vi "tls http connection handler.vi"(8 "http responder":refnum<class "https responder.lvclass">, 9 "remote address":string, 10 "basic HTTP handler dataset":refnum<class "HTTPS handler dataset.lvclass">, 11 "connection":refnum<k5>) -> ()   [LabVIEW 2016, in "Basic HTTPS server.lvclass"]
uses:
  Basic HTTPS server.lvclass
  HTTP responder/https responder.lvclass
  HTTP handler dataset/HTTPS handler dataset.lvclass
  HTTP handler dataset/HTTPS handler dataset.lvclass/HTTPS handler dataset.ctl
  http request.ctl
  http method.ctl
  HTTP headers/http header data.ctl
  https handler parse state.ctl
  HTTP headers/http headers.lvlib
  lvlibtls/socket connection/lvlibretls connection.lvclass
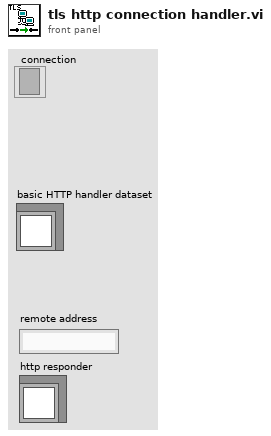
[diagram p1: front panel]
types:
  T1 = typedef "Basic HTTPS server.lvclass/http server info.ctl" = cluster{"port":u16}
  T2 = typedef "Basic HTTPS server.lvclass/http server properties.ctl" = cluster{"max url size":i32, "max header":i32, "timeout ms":i32, "max data size":i32}
  T3 = typedef "Basic HTTPS server.lvclass/https handler parse state.ctl" = enum16{"function", "headers", "data", "process"}
  T4 = typedef "Basic HTTPS server.lvclass/http request.ctl" = cluster{"type":T5, "remote address":string, "method":string, "url":string, "version":string, "headers":T6, "data":string}
  T5 = typedef "Basic HTTPS server.lvclass/http method.ctl" = enum16{"application", "error", "upgrade"}
  T6 = typedef "http headers.lvlib/http header data.ctl" = cluster{"lookup":variant}
  T7 = typedef "Basic HTTPS server.lvclass/http response.ctl" = cluster{"reason code":u16, "status string":string, "headers":T6, "cookies":string[], "data":string}
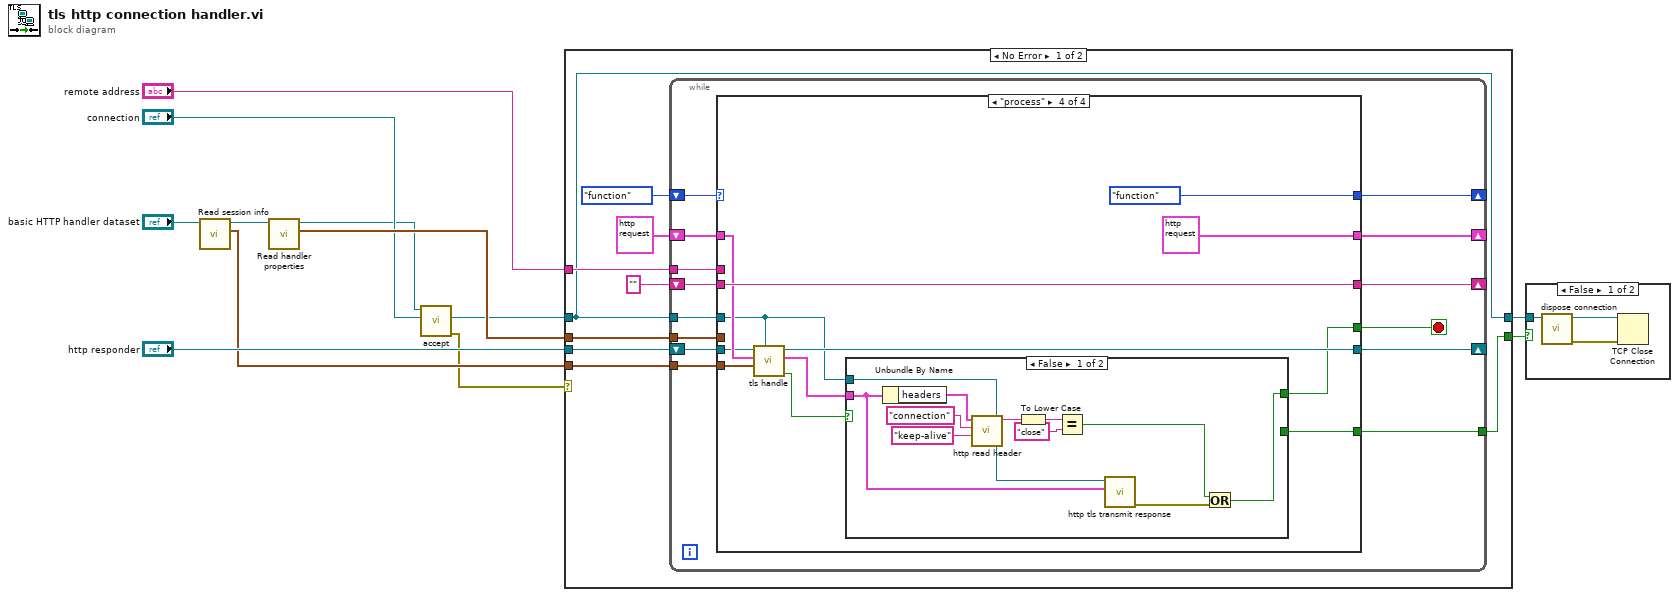
[diagram p0: block diagram]
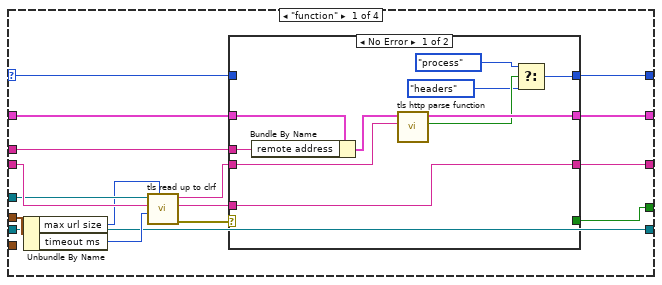
[diagram p2: hidden frame]
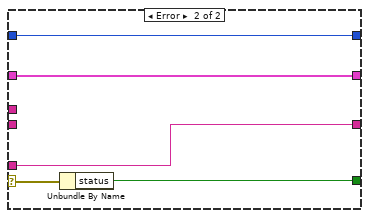
[diagram p3: hidden frame]
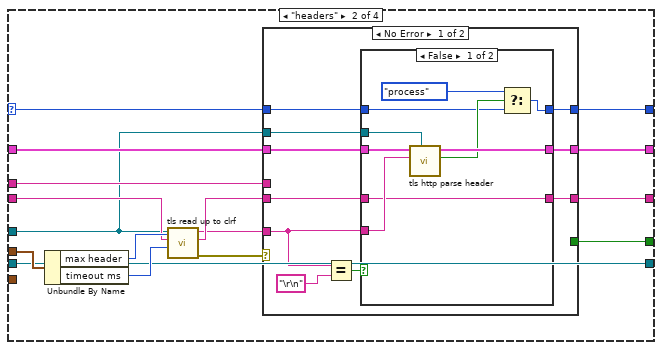
[diagram p4: hidden frame]
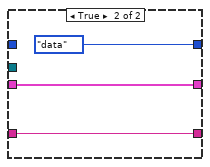
[diagram p5: hidden frame]
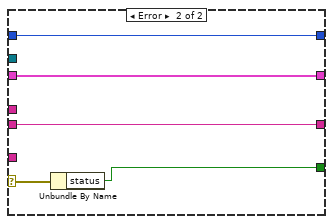
[diagram p6: hidden frame]
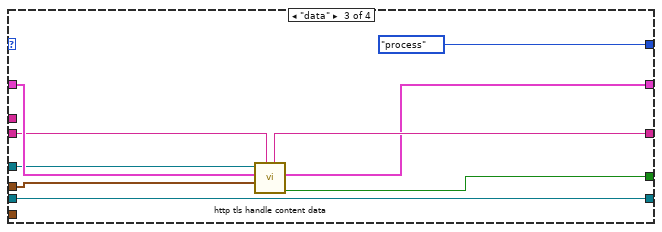
[diagram p7: hidden frame]
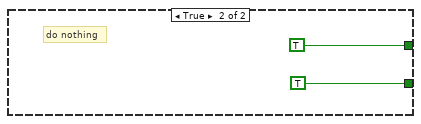
[diagram p8: hidden frame]
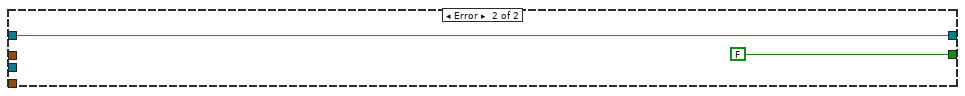
[diagram p9: hidden frame]
diagram:
  n1 = call "Read session info.vi"("basic HTTP handler dataset in"="basic HTTP handler dataset") -> ("server information"=w7:T1, "basic HTTP handler dataset out"=w9:refnum<class "HTTPS handler dataset.lvclass">)  [unwired: 9 in]
  n2 = call "Read handler properties.vi"("basic HTTP handler dataset in"=w9) -> ("server properties"=w10:T2, "basic HTTP handler dataset out"=w1:refnum<class "HTTPS handler dataset.lvclass">)  [unwired: 9 in]
  n3 = call "accept.vi"("connection ID"="connection", "TLS HTTP handler dataset in"=w1) -> ("error out"=w6:errorcluster, "lvlibretls connection"=w5:refnum<class "lvlibretls connection.lvclass">)  [unwired: 8 in]
  n4 = case shown="No Error" w6 {
    tunnel: w5 -> [w17 w145]
    tunnel: "remote address" -> [w21 _]
    tunnel: w10 -> [w19 _]
    tunnel: "http responder" -> [w14 _]
    tunnel: w7 -> [w15 _]
    tunnel: [w17 w145] -> w3
    tunnel: [w13 FALSE] -> w2
    frame No Error {
      n5 = while {
        tunnel: w17 -> [w28]
        shift-right: [w34] -> _
        shift-left: T4 {"type"=enum."application", "remote address"="", "method"="", "url"="", "version"="", "headers"={"lookup"=variant}, "data"=""} ("application request") -> [w35]
        shift-right: [w33] -> _
        shift-left: https_handler_parse_state."function" -> [w30]
        tunnel: w21 -> [w32]
        tunnel: w19 -> [w31]
        shift-right: [w26] -> _
        shift-left: "" -> [w27]
        tunnel: w15 -> [w25]
        shift-right: [w23] -> _
        shift-left: w14 -> [w24]
        tunnel: [w22] -> w13
        stop <- w29 stop-if-true
        n6 = case shown="\"process\"" w30 {
          selector: w30 -> [w47 w78 _ _]
          tunnel: w35 -> [w51 w82 w117 w126]
          tunnel: [w50 w81 w111 T4 {"type"=enum."application", "remote address"="", "method"="", "url"="", "version"="", "headers"={"lookup"=variant}, "data"=""} ("application request")] -> w34
          tunnel: w28 -> [w43 w68 w116 w122]
          tunnel: [w49 w80 https_handler_parse_state."process" https_handler_parse_state."function"] -> w33
          tunnel: w32 -> [w48 w79 _ _]
          tunnel: w31 -> [w46 w77 w118 _]
          tunnel: [w36 w67 w110 w120] -> w29
          tunnel: w27 -> [w45 w73 w115 w128]
          tunnel: [w38 w76 w114 w128] -> w26
          tunnel: w25 -> [_ _ _ w127]
          tunnel: w24 -> [w37 w69 w112 w125]
          tunnel: [w37 w69 w112 w124] -> w23
          tunnel: [_ _ _ w119] -> w22
          frame "function" {
            n7 = Unbundle By Name(w46) -> ("max url size"=w41:i32, "timeout ms"=w42:i32)
            n8 = call "tls read up to clrf.vi"("max size"=w41, "timeout ms"=w42, "buffer in"=w45, "lvlibretls connection in"=w43) -> ("error out"=w40:errorcluster, "buffer out"=w39:string, "line out"=w44:string)  [unwired: 5 in]
            n9 = case shown="No Error" w40 {
              selector: w40 -> [_ w65]
              tunnel: w51 -> [w60 w66]
              tunnel: [w61 w66] -> w50
              tunnel: w39 -> [w57 w63]
              tunnel: w47 -> [_ w64]
              tunnel: [w52 w64] -> w49
              tunnel: w48 -> [w59 _]
              tunnel: w44 -> [w56 _]
              tunnel: [w57 w63] -> w38
              tunnel: [_ w62] -> w36
              frame No Error {
                n10 = Bundle By Name(cluster=w60, "remote address"=w59) -> (w58:T4)
                n11 = call "tls http parse function.vi"("data in"=w56, "application request in"=w58) -> ("error"=w55:bool, "application request out"=w61:T4)  [unwired: 8 in]
                n12 = Select(t=https_handler_parse_state."process", s=w55, f=https_handler_parse_state."headers") -> (s? t:f=w52:T3)
              }
              frame Error {
                n13 = Unbundle By Name(w65) -> ("status"=w62:bool)
              }
            }
          }
          frame "headers" {
            n14 = Unbundle By Name(w77) -> ("max header"=w75:i32, "timeout ms"=w74:i32)
            n15 = call "tls read up to clrf.vi"("max size"=w75, "timeout ms"=w74, "buffer in"=w73, "lvlibretls connection in"=w68) -> ("error out"=w70:errorcluster, "buffer out"=w72:string, "line out"=w71:string)  [unwired: 5 in]
            n16 = case shown="No Error" w70 {
              selector: w70 -> [_ w108]
              tunnel: w82 -> [w88 w109]
              tunnel: [w89 w109] -> w81
              tunnel: w71 -> [w91 _]
              tunnel: w78 -> [w92 w107]
              tunnel: [w90 w107] -> w80
              tunnel: w79 -> [_ _]
              tunnel: w72 -> [w84 w106]
              tunnel: [w85 w106] -> w76
              tunnel: w68 -> [w83 _]
              tunnel: [_ w105] -> w67
              frame No Error {
                n17 = Equal?(x=w91, y="\r\n" ("x")) -> (x = y?=w86:bool)
                n18 = case shown="False" w86 {
                  tunnel: w91 -> [w101 _]
                  tunnel: w88 -> [w100 w104]
                  tunnel: [w99 w104] -> w89
                  tunnel: w92 -> [w96 _]
                  tunnel: [w95 https_handler_parse_state."data"] -> w90
                  tunnel: [w98 w103] -> w85
                  tunnel: w84 -> [w98 w103]
                  tunnel: w83 -> [w93 _]
                  frame False {
                    n19 = call "tls http parse header.vi"("lvlibretls connection in"=w93, "data in"=w101, "application request"=w100) -> ("abort"=w97:bool, "application request out"=w99:T4)  [unwired: 7 in]
                    n20 = Select(t=https_handler_parse_state."process", s=w97, f=w96) -> (s? t:f=w95:T3)
                  }
                  frame True {
                  }
                }
              }
              frame Error {
                n21 = Unbundle By Name(w108) -> ("status"=w105:bool)
              }
            }
          }
          frame "data" {
            n22 = call "http tls handle content data.vi"("buffer in"=w115, "server properties"=w118, "application request"=w117, "lvlibretls connection in"=w116) -> ("connection error"=w110:bool, "application request out"=w111:T4, "buffer out"=w114:string)  [unwired: 5 in]
          }
          frame "process" {
            n23 = call "tls handle.vi"("lvlibretls connection"=w122, "server information"=w127, "application request in"=w126, "http responder in"=w125) -> ("connection upgrade"=w121:bool, "response"=w123:T7, "http responder out"=w124:refnum<class "https responder.lvclass">)  [unwired: 5 in]
            n24 = case shown="False" w121 {
              tunnel: w123 -> [w135 _]
              tunnel: w122 -> [w136 _]
              tunnel: [w132 TRUE] -> w120
              tunnel: [_ TRUE] -> w119
              frame False {
                n25 = Unbundle By Name(w135) -> ("headers"=w140:T6)
                n26 = call "http read header.vi"("default value"="keep-alive", "header field name"="connection" ("name"), "headers"=w140) -> ("value"=w137:string)  [unwired: 7 in, 1 out]
                n27 = To Lower Case(string=w137) -> (all lower case string=w131:string)
                n28 = Equal?(x=w131, y="close" ("name")) -> (x = y?=w133:bool)
                n29 = call "http tls transmit response.vi"("application request"=w135, "lvlibretls connection in"=w136) -> ("error out"=w134:errorcluster)  [unwired: 9 in]
                n30 = Or(x=w133, y=w134) -> (x .or. y?=w132:bool)
              }
              frame True {
                # "do nothing"
              }
            }
          }
        }
      }
    }
    frame Error {
    }
  }
  n31 = case shown="False" w2 {
    tunnel: w3 -> [w148 _]
    frame False {
      n32 = call "dispose connection.vi"("lvlibretls connection in"=w148) -> ("error out"=w146:errorcluster, "connection"=w147:refnum<k5>)  [unwired: 9 in]
      n33 = TCP Close Connection(connection ID=w147, error in (no error)=w146) -> ()  [unwired: 1 in, 2 out]
    }
    frame True {
    }
  }
